vi "GVSResize Panel Child.vi"(8 "spliter array":refnum<vi>[](array[refnum]), 9 "SubPanel array":refnum<vi>[](array[refnum]), 10 "DataView Array Idx":i32) -> ()   [LabVIEW 2013]
uses:
  GVSNew View Global.vi
panel:
  in  "cur_sp_hei":i32
  in  "cur_sp_wid":i32
  in  "cur_sp_ypos":i32
  in  "cur_sp_xpos":i32
  in  "sp_mUp_hei":i32
  in  "sp_mUp_wid":i32
  in  "sp_mUp_ypos":i32
  in  "sp_mUp_xpos":i32
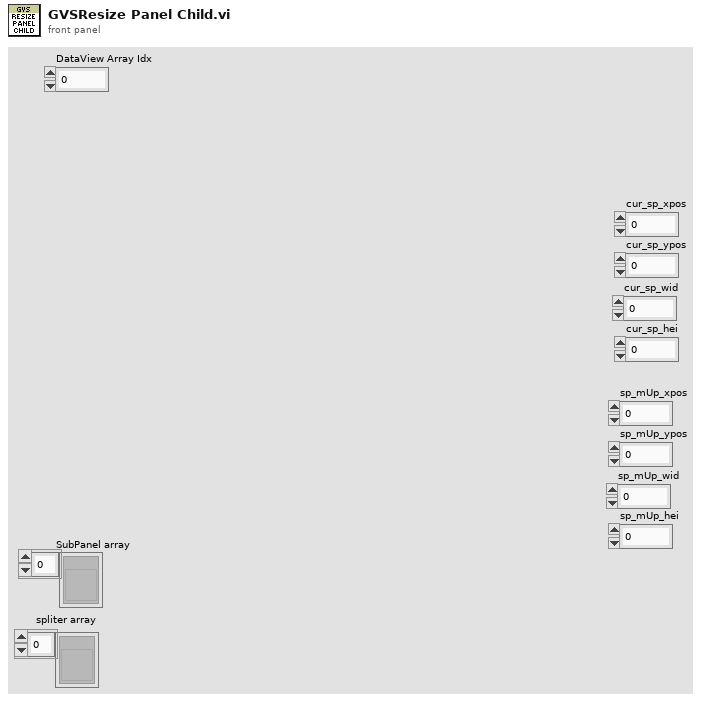
[diagram p1: front panel]
types:
  T1 = typedef "Graph Main Info Cluster.ctl" = cluster{"Selected_BarIdx":i32, "Selected_PanelIdx":i32, "Graph Main VIRef":refnum<vi>, "ToolBarClick":bool, "Spliter Ref Array":refnum<vi>[], "Panel Ref Array":refnum<vi>[], "Spliter_matrix":i32[][], "Panel_matrix":i32[][], "child_spliterIdx_matrix":i32[][], "split_pos_matrix":i32[][], "Title State":bool, "sQueueName":string, "Frame nID":i32, "Graph VIRef Array":cluster{"Graph VIRef":refnum<vi>, "Panel Idx":i32, "Frame VIRef":refnum<vi>, "Icon Ring":i32, "Graph Type":string}[], "View Type":string}
  T2 = typedef "LVPositionTypeDef.ctl" = cluster{"Left":i32, "Top":i32}
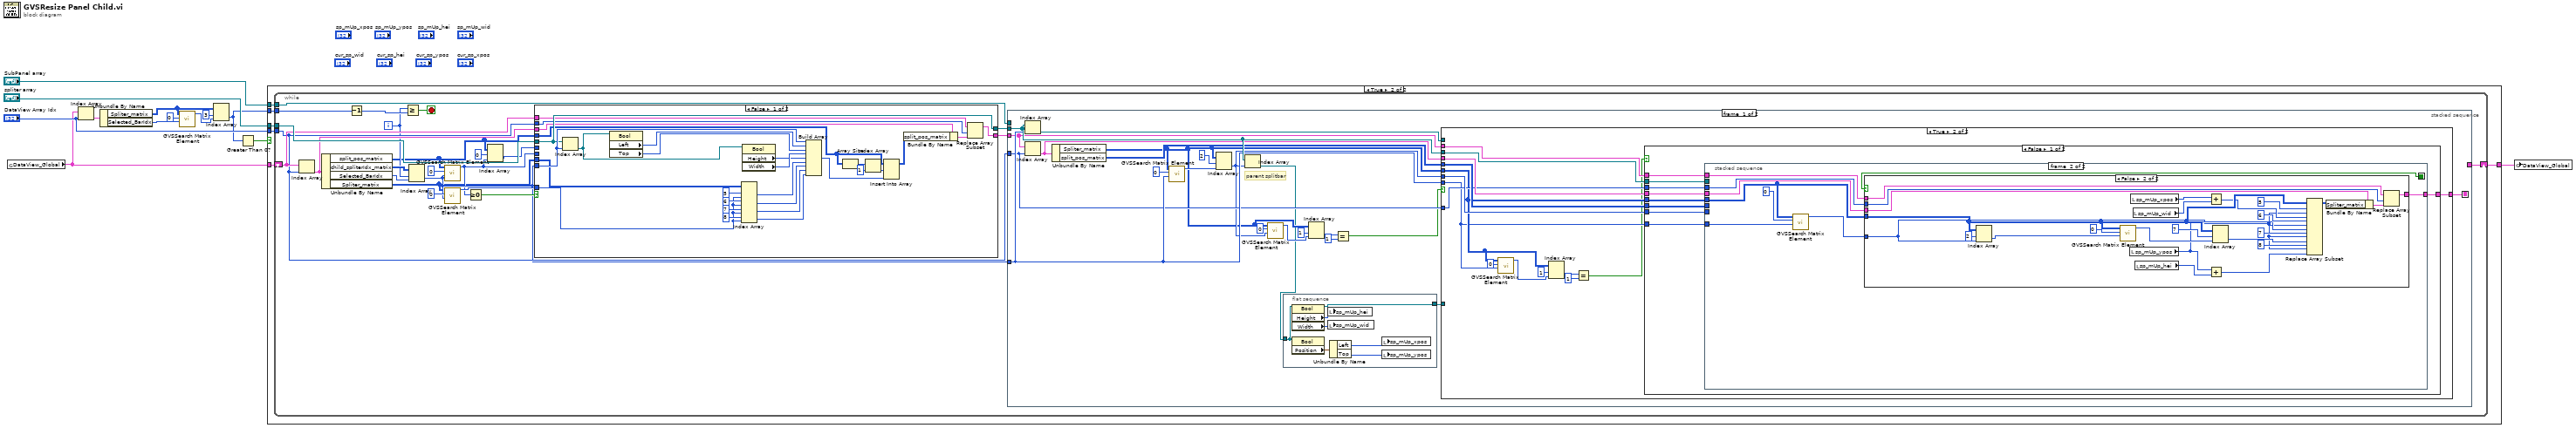
[diagram p0: block diagram]
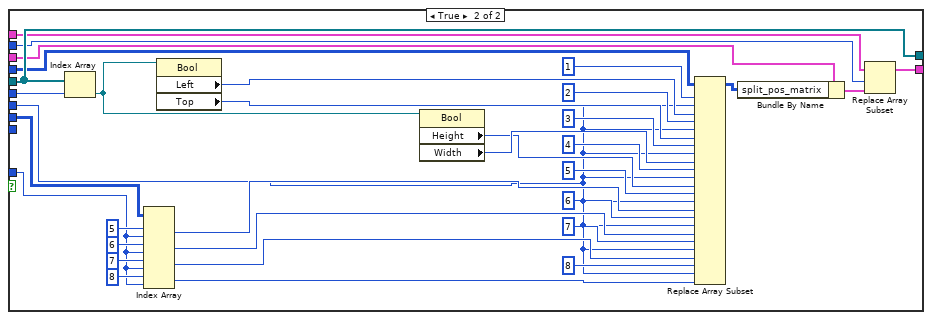
[diagram p3: hidden frame]
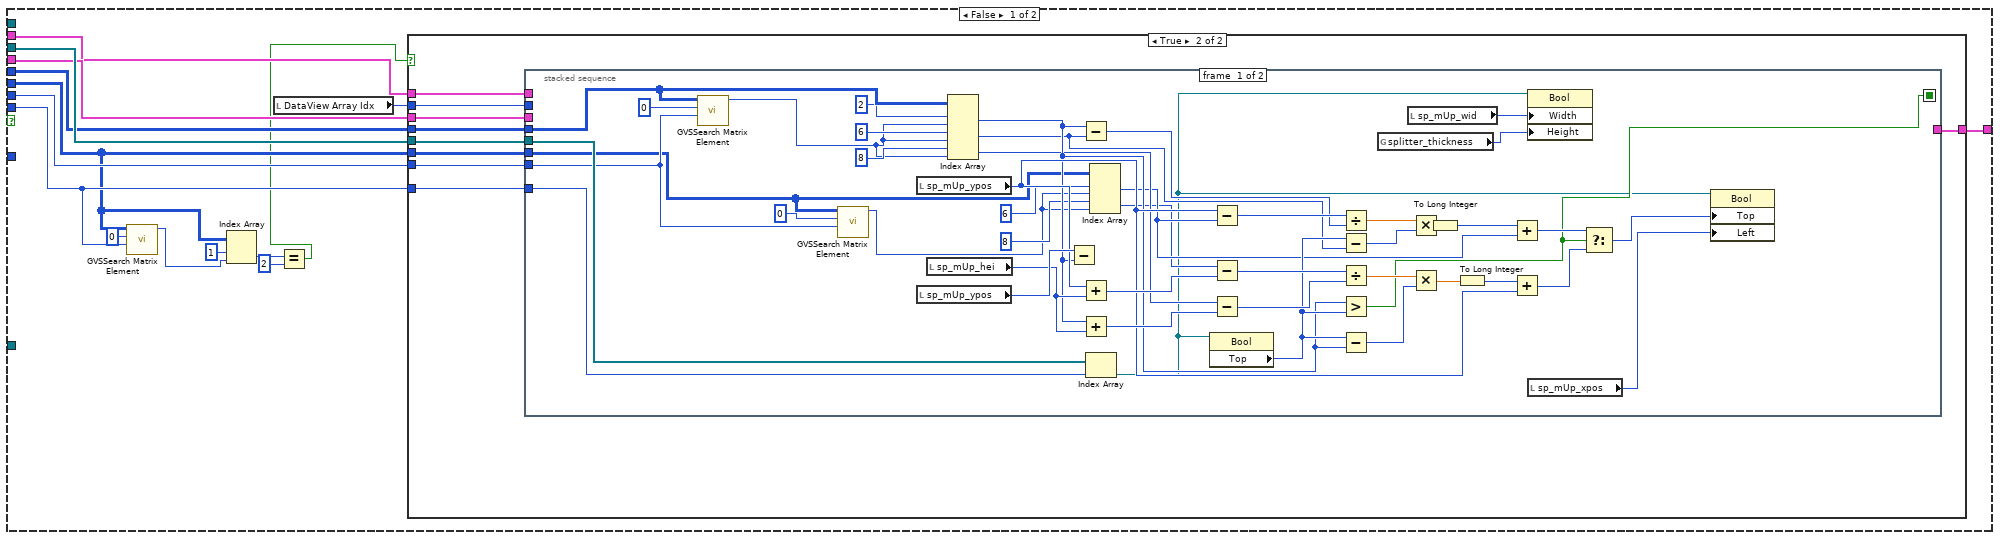
[diagram p4: hidden frame]
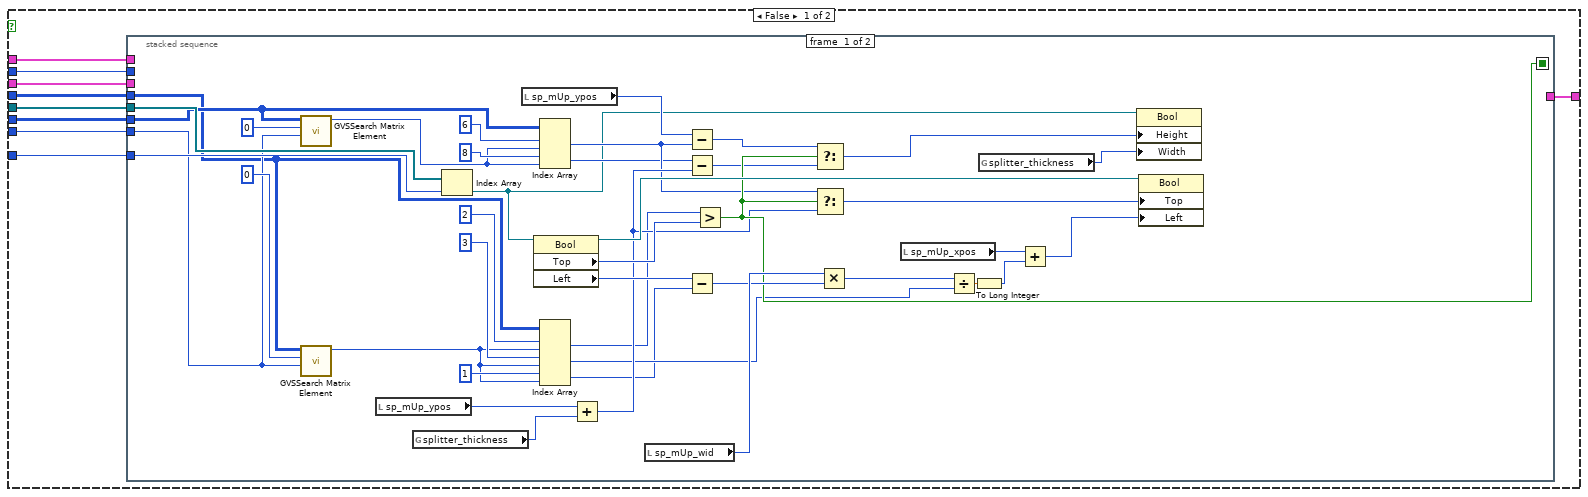
[diagram p5: hidden frame]
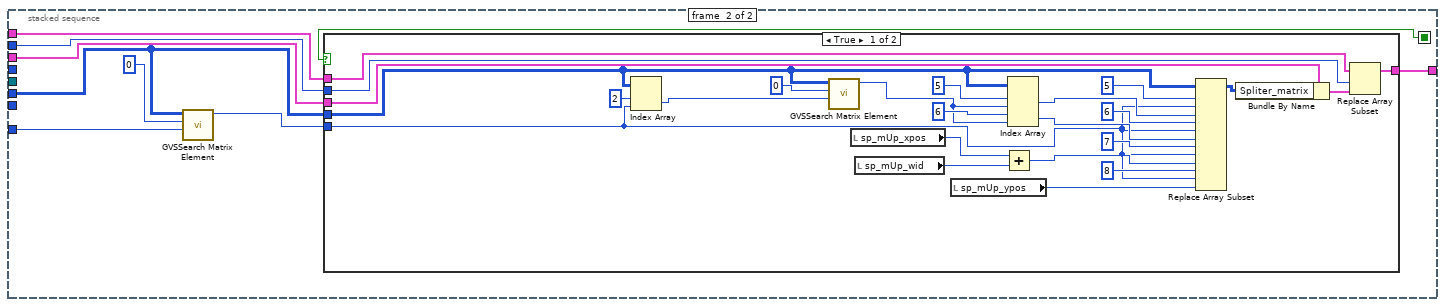
[diagram p6: hidden frame]
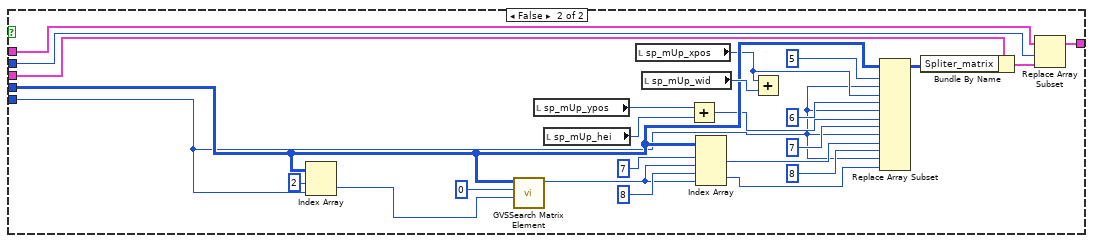
[diagram p7: hidden frame]
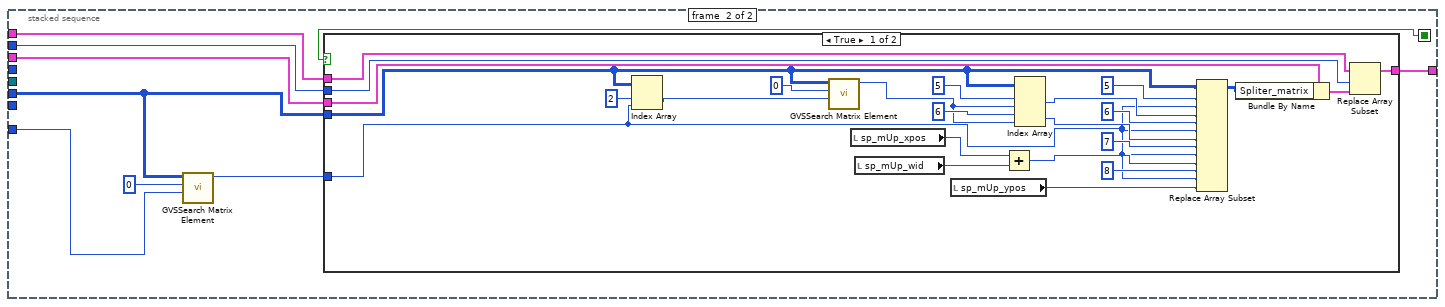
[diagram p8: hidden frame]
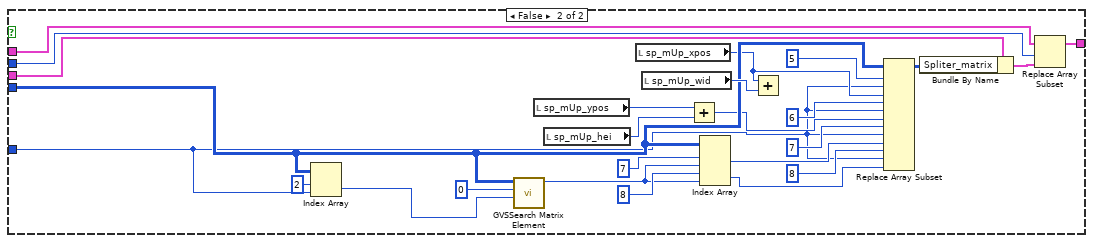
[diagram p9: hidden frame]
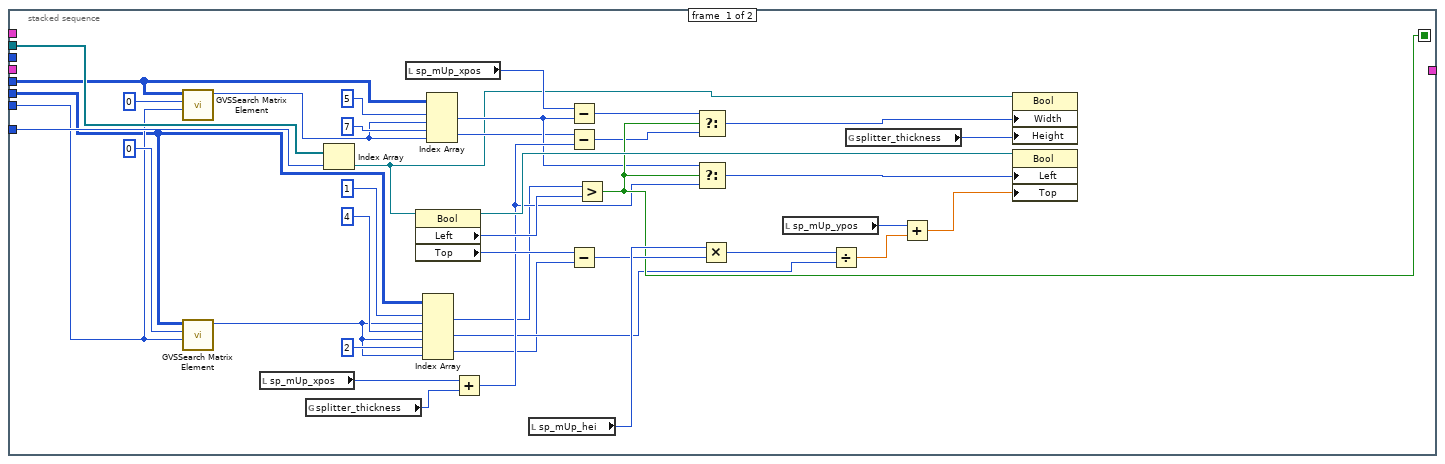
[diagram p10: hidden frame]
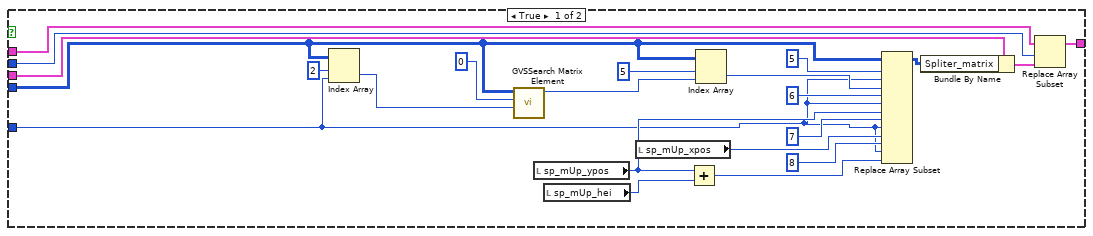
[diagram p11: hidden frame]
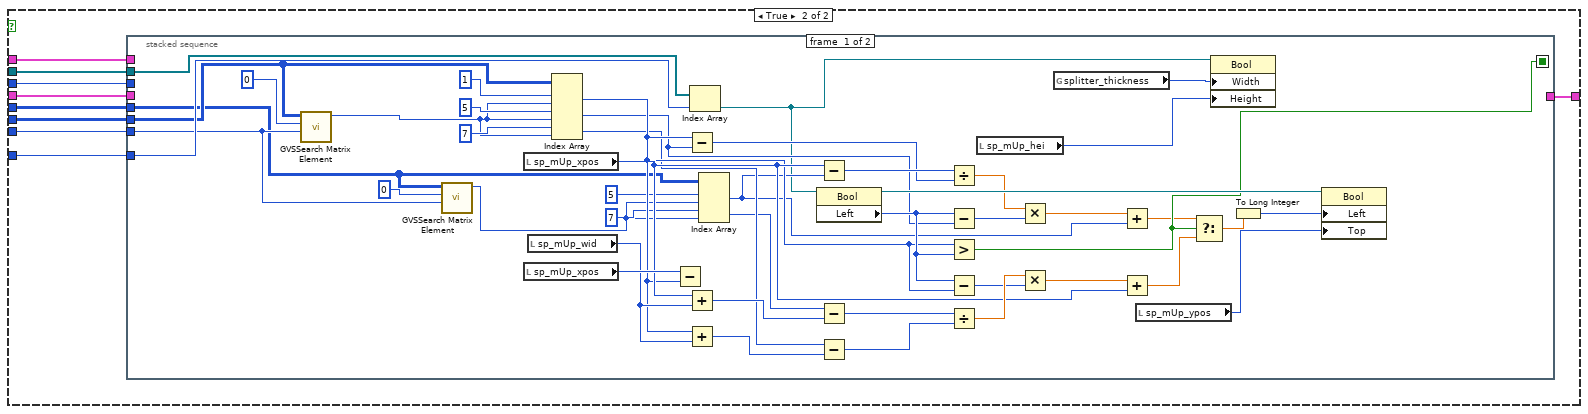
[diagram p12: hidden frame]
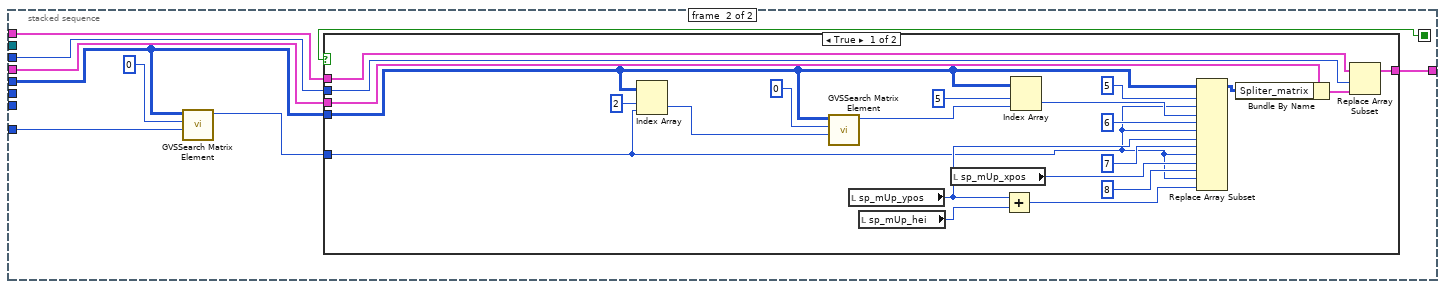
[diagram p13: hidden frame]
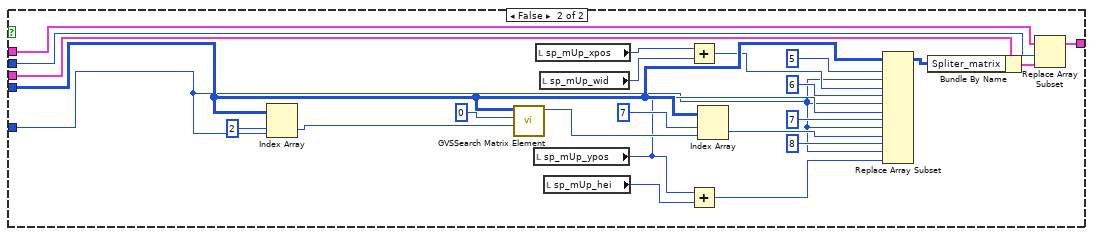
[diagram p14: hidden frame]
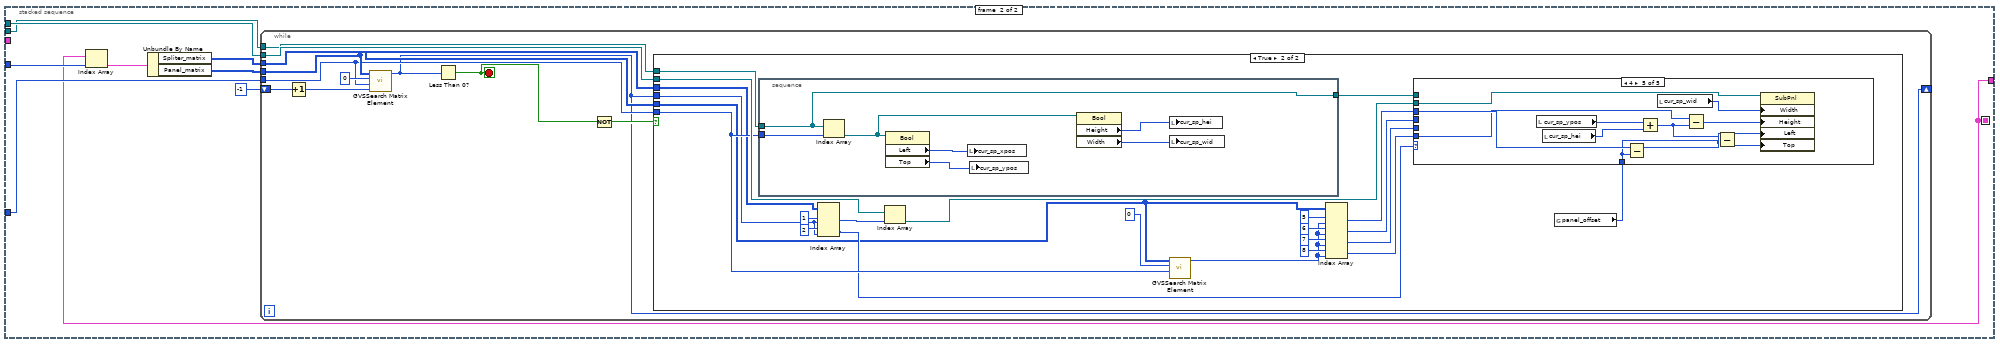
[diagram p15: hidden frame]
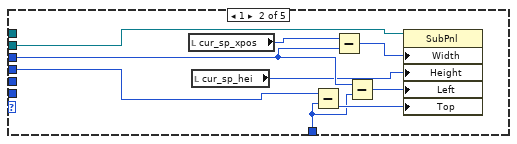
[diagram p18: hidden frame]
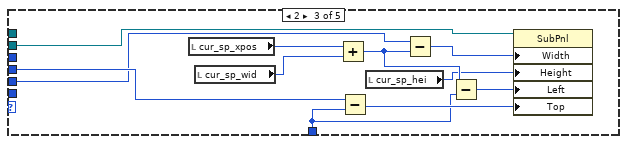
[diagram p19: hidden frame]
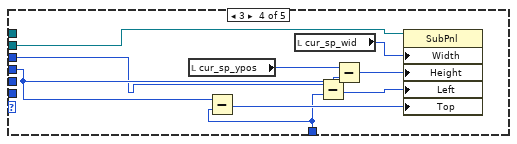
[diagram p20: hidden frame]
diagram:
  n1 = global read "GVSNew View Global.vi" "DataView_Global"() -> (w7:T1[])
  n2 = Index Array(array=w7, index="DataView Array Idx") -> (element=w10:T1)
  n3 = Unbundle By Name(w10) -> ("Spliter_matrix"=w4:i32[][], "Selected_BarIdx"=w9:i32)
  n4 = call "GVSSearch Matrix Element.vi"("element"=w9, "index (row)"=0, "matrix in"=w4) -> ("index of element"=w2:i32)  [unwired: 8 in]
  n5 = Index Array(array=w4, index (row)=3, index (col)=w2) -> (element=w1:i32)
  n6 = Greater Than 0?(x=w1) -> (x > 0?=w5:bool)
  n7 = case shown="True" w5 {
    tunnel: "spliter array" -> [_ w20]
    tunnel: "SubPanel array" -> [_ w19]
    tunnel: "DataView Array Idx" -> [_ w18]
    tunnel: w1 -> [_ w17]
    tunnel: w7 -> [w14 w16]
    tunnel: [w14 w15] -> w6
    frame False {
    }
    frame True {
      n8 = while {
        tunnel: w20 -> [w41]
        tunnel: w17 -> [w30]
        tunnel: w19 -> [w39]
        tunnel: w18 -> [w31]
        shift-right: [w32] -> w15
        shift-left: w16 -> [w34]
        i -> [w28]
        stop <- w42 stop-if-true
        n9 = Index Array(array=w34, index=w31) -> (element=w38:T1)
        n10 = Unbundle By Name(w38) -> ("split_pos_matrix"=w24:i32[][], "child_spliterIdx_matrix"=w29:i32[][], "Selected_BarIdx"=w27:i32, "Spliter_matrix"=w21:i32[][])
        n11 = Decrement(x=w30) -> (x-1=w43:i32)
        n12 = Greater Or Equal?(x=w28, y=w43) -> (x >= y?=w42:bool)
        n13 = Index Array(array=w29, index (row)=w28, index (col)=w27) -> (element=w26:i32)
        n14 = call "GVSSearch Matrix Element.vi"("element"=w26, "index (row)"=0, "matrix in"=w24) -> ("index of element"=w23:i32)  [unwired: 8 in]
        n15 = call "GVSSearch Matrix Element.vi"("element"=w26, "index (row)"=0, "matrix in"=w21) -> ("index of element"=w36:i32)  [unwired: 8 in]
        n16 = Greater Or Equal To 0?(x=w23) -> (x >= 0?=w44:bool)
        n17 = Index Array(array=w24, index (row)=0, index (col)=w23) -> (element=w22:i32)
        n18 = case shown="False" w44 {
          tunnel: w23 -> [_ w76]
          tunnel: w26 -> [w72 _]
          tunnel: w41 -> [w67 w104]
          tunnel: w22 -> [_ w105]
          tunnel: [w67 w104] -> w40
          tunnel: w36 -> [w57 w93]
          tunnel: w21 -> [w56 w94]
          tunnel: w24 -> [w48 w92]
          tunnel: w31 -> [w65 w102]
          tunnel: w38 -> [w64 w101]
          tunnel: w34 -> [w63 w100]
          tunnel: [w62 w99] -> w33
          frame False {
            n19 = Index Array(array=w67, index=w72) -> (element=w45:refnum<vi>)
            n20 = property class="Bool"(reference=w45) -> ("Left"=w71:i32, "Top"=w70:i32)  [unwired: 1 in, 2 out]
            n21 = Index Array(array=w56, index (row) #1=5 ("index (row)"), index (col) #1=w57, index (row) #2=6 ("index (row)"), index (col) #2=w57, index (row) #3=7 ("index (row)"), index (col) #3=w57, index (row) #4=8 ("index (row)"), index (col) #4=w57) -> (element #1=w55:i32, element #2=w54:i32, element #3=w53:i32, element #4=w52:i32)
            n22 = property class="Bool"(reference=w45) -> ("Height"=w68:u32, "Width"=w69:u32)  [unwired: 1 in, 2 out]
            n23 = Build Array(w72, w71, w70, w69, w68, w55, w54, w53, w52) -> (w47:u32[])
            n24 = Array Size(array=w48) -> (size(s)=w51:i32[])
            n25 = Index Array(array=w51, index=1) -> (element=w49:i32)
            n26 = Insert Into Array(array=w48, index (col)=w49, new element=w47) -> (w46:i32[][])  [unwired: 1 in]
            n27 = Bundle By Name(cluster=w64, "split_pos_matrix"=w46) -> (w66:T1)
            n28 = Replace Array Subset(array=w63, new element=w66, index=w65) -> (w62:T1[])
          }
          frame True {
            n29 = Index Array(array=w104, index=w105) -> (element=w73:refnum<vi>)
            n30 = Index Array(array=w94, index (row) #1=5 ("index (row)"), index (col) #1=w93, index (row) #2=6 ("index (row)"), index (col) #2=w93, index (row) #3=7 ("index (row)"), index (col) #3=w93, index (row) #4=8 ("index (row)"), index (col) #4=w93) -> (element #1=w82:i32, element #2=w80:i32, element #3=w78:i32, element #4=w75:i32)
            n31 = property class="Bool"(reference=w73) -> ("Left"=w90:i32, "Top"=w88:i32)  [unwired: 1 in, 2 out]
            n32 = property class="Bool"(reference=w73) -> ("Height"=w84:u32, "Width"=w86:u32)  [unwired: 1 in, 2 out]
            n33 = Replace Array Subset(array=w92, new element #1=w90, index (row) #1=1 ("disabled index (row)"), index (col) #1=w76, new element #2=w88, index (row) #2=2 ("disabled index (row)"), index (col) #2=w76, new element #3=w86, index (row) #3=3 ("disabled index (row)"), index (col) #3=w76, new element #4=w84, index (row) #4=4 ("disabled index (row)"), index (col) #4=w76, new element #5=w82, index (row) #5=5 ("disabled index (row)"), index (col) #5=w76, new element #6=w80, index (row) #6=6 ("disabled index (row)"), index (col) #6=w76, new element #7=w78, index (row) #7=7 ("disabled index (row)"), index (col) #7=w76, new element #8=w75, index (row) #8=8 ("disabled index (row)"), index (col) #8=w76) -> (w74:i32[][])
            n34 = Bundle By Name(cluster=w101, "split_pos_matrix"=w74) -> (w103:T1)
            n35 = Replace Array Subset(array=w100, new element=w103, index=w102) -> (w99:T1[])
          }
        }
        n36 = stacked-sequence {
          seq-local: [w119 _] -> [_ w595]
          tunnel: w40 -> [w125 w601]
          tunnel: w26 -> [w121 w603]
          tunnel: w39 -> [_ w602]
          tunnel: w31 -> [w118 w598]
          tunnel: w33 -> [w120 _]
          tunnel: [_ w595] -> w32
          frame #0 {
            # "parent splitbar"
            n37 = Index Array(array=w125, index=w121) -> (element=w126:refnum<vi>)
            n38 = Index Array(array=w120, index=w118) -> (element=w123:T1)
            n39 = Unbundle By Name(w123) -> ("Spliter_matrix"=w113:i32[][], "split_pos_matrix"=w124:i32[][])
            n40 = call "GVSSearch Matrix Element.vi"("element"=w121, "index (row)"=0, "matrix in"=w113) -> ("index of element"=w116:i32)  [unwired: 8 in]
            n41 = Index Array(array=w113, index (row)=2, index (col)=w116) -> (element=w114:i32)
            n42 = Index Array(array=w125, index=w114) -> (element=w107:refnum<vi>)
            n43 = call "GVSSearch Matrix Element.vi"("element"=w114, "index (row)"=0, "matrix in"=w113) -> ("index of element"=w111:i32)  [unwired: 8 in]
            n44 = flat-sequence {
              tunnel: w107 -> [w128]
              tunnel: [w127] -> w106
              frame #0 {
                n45 = property class="Bool"(reference=w128) -> (reference out=w127:refnum<vi>, "Height"=w130:u32, "Width"=w129:u32)  [unwired: 1 in, 1 out]
                n46 = property class="Bool"(reference=w128) -> ("Position"=w133:T2)  [unwired: 1 in, 2 out]
                n47 = local write "sp_mUp_hei"(w130) -> ()
                n48 = local write "sp_mUp_wid"(w129) -> ()
                n49 = Unbundle By Name(w133) -> ("Left"=w132:i32, "Top"=w131:i32)
                n50 = local write "sp_mUp_xpos"(w132) -> ()
                n51 = local write "sp_mUp_ypos"(w131) -> ()
              }
            }
            n52 = Index Array(array=w113, index (row)=1, index (col)=w111) -> (element=w110:i32)
            n53 = Equal?(x=w110, y=1) -> (x = y?=w108:bool)
            n54 = case shown="True" w108 {
              tunnel: w126 -> [_ _]
              tunnel: w114 -> [w148 w382]
              tunnel: w125 -> [w147 w381]
              tunnel: w121 -> [w141 w369]
              tunnel: w124 -> [w146 w380]
              tunnel: w113 -> [w136 w370]
              tunnel: w123 -> [w145 w379]
              tunnel: w120 -> [w143 w378]
              tunnel: [w142 w377] -> w119
              tunnel: w118 -> [_ w376]
              tunnel: w106 -> [_ _]
              frame False {
                n55 = call "GVSSearch Matrix Element.vi"("element"=w141, "index (row)"=0, "matrix in"=w136) -> ("index of element"=w135:i32)  [unwired: 8 in]
                n56 = Index Array(array=w136, index (row)=1, index (col)=w135) -> (element=w138:i32)
                n57 = local read "DataView Array Idx"() -> (w144:i32)
                n58 = Equal?(x=w138, y=2) -> (x = y?=w134:bool)
                n59 = case shown="True" w134 {
                  tunnel: w148 -> [w155 w262]
                  tunnel: w147 -> [w157 w263]
                  tunnel: w141 -> [w156 w264]
                  tunnel: w146 -> [w154 w261]
                  tunnel: w136 -> [w153 w260]
                  tunnel: w145 -> [w152 w259]
                  tunnel: w144 -> [w151 w258]
                  tunnel: w143 -> [w150 w257]
                  tunnel: [w149 w256] -> w142
                  frame False {
                    n60 = stacked-sequence {
                      seq-local: [w184 _] -> [_ w206]
                      tunnel: w157 -> [w196 _]
                      tunnel: w156 -> [w195 w201]
                      tunnel: w155 -> [w176 _]
                      tunnel: w154 -> [w169 _]
                      tunnel: w153 -> [w175 w203]
                      tunnel: w152 -> [_ w205]
                      tunnel: w151 -> [_ w204]
                      tunnel: w150 -> [_ w199]
                      tunnel: [_ w198] -> w149
                      frame #0 {
                        n61 = call "GVSSearch Matrix Element.vi"("element"=w176, "index (row)"=0, "matrix in"=w175) -> ("index of element"=w172:i32)  [unwired: 8 in]
                        n62 = call "GVSSearch Matrix Element.vi"("element"=w176, "index (row)"=0, "matrix in"=w169) -> ("index of element"=w165:i32)  [unwired: 8 in]
                        n63 = local read "sp_mUp_ypos"() -> (w194:i32)
                        n64 = global read "GVSNew View Global.vi" "splitter_thickness"() -> (w158:u32)
                        n65 = Index Array(array=w196, index=w195) -> (element=w161:refnum<vi>)
                        n66 = local read "sp_mUp_ypos"() -> (w182:i32)
                        n67 = property class="Bool"(reference=w161) -> (reference out=w197:refnum<vi>, "Top"=w183:i32, "Left"=w186:i32)  [unwired: 1 in, 1 out]
                        n68 = Index Array(array=w175, index (row) #1=6 ("index (row)"), index (col) #1=w172, index (row) #2=8 ("index (row)"), index (col) #2=w172) -> (element #1=w171:i32, element #2=w170:i32)
                        n69 = Index Array(array=w169, index (row) #1=2 ("index (row)"), index (col) #1=w165, index (row) #2=3 ("index (row)"), index (col) #2=w165, index (row) #3=1 ("index (row)"), index (col) #3=w165) -> (element #1=w164:i32, element #2=w163:i32, element #3=w162:i32)
                        n70 = Add(x=w194, y=w158) -> (x+y=w180:u32)
                        n71 = local read "sp_mUp_wid"() -> (w191:i32)
                        n72 = Subtract(x=w182, y=w171) -> (x-y=w181:i32)
                        n73 = Subtract(x=w170, y=w180) -> (x-y=w179:u32)
                        n74 = Subtract(x=w186, y=w162) -> (x-y=w185:i32)
                        n75 = Greater?(x=w164, y=w183) -> (0:w184:bool)
                        n76 = Select(t=w181, s=w184, f=w179) -> (s? t:f=w192:u32)
                        n77 = Select(t=w171, s=w184, f=w180) -> (s? t:f=w193:u32)
                        n78 = Multiply(x=w191, y=w185) -> (x*y=w190:i32)
                        n79 = local read "sp_mUp_xpos"() -> (w189:i32)
                        n80 = Divide(x=w190, y=w163) -> (x/y=w188:dbl)
                        n81 = To Long Integer(number=w188) -> (32bit integer=w160:i32)
                        n82 = global read "GVSNew View Global.vi" "splitter_thickness"() -> (w159:u32)
                        n83 = Add(x=w189, y=w160) -> (x+y=w187:i32)
                        n84 = property class="Bool"(reference=w161, "Height"=w192, "Width"=w159) -> ()  [unwired: 1 in, 2 out]
                        n85 = property class="Bool"(reference=w197, "Top"=w193, "Left"=w187) -> ()  [unwired: 1 in, 2 out]
                      }
                      frame #1 {
                        n86 = call "GVSSearch Matrix Element.vi"("element"=w201, "index (row)"=0, "matrix in"=w203) -> ("index of element"=w200:i32)  [unwired: 8 in]
                        n87 = case shown="True" w206 {
                          tunnel: w200 -> [w209 w233]
                          tunnel: w203 -> [w217 w241]
                          tunnel: w205 -> [w227 w251]
                          tunnel: w204 -> [w226 w250]
                          tunnel: w199 -> [w224 w248]
                          tunnel: [w223 w247] -> w198
                          frame True {
                            n88 = Index Array(array=w217, index (row)=2, index (col)=w209) -> (element=w221:i32)
                            n89 = call "GVSSearch Matrix Element.vi"("element"=w221, "index (row)"=0, "matrix in"=w217) -> ("index of element"=w218:i32)  [unwired: 8 in]
                            n90 = local read "sp_mUp_xpos"() -> (w229:i32)
                            n91 = local read "sp_mUp_wid"() -> (w230:i32)
                            n92 = local read "sp_mUp_ypos"() -> (w208:i32)
                            n93 = Add(x=w229, y=w230) -> (x+y=w211:i32)
                            n94 = Index Array(array=w217, index (row) #1=5 ("index (row)"), index (col) #1=w218, index (row) #2=6 ("index (row)"), index (col) #2=w218) -> (element #1=w215:i32, element #2=w213:i32)
                            n95 = Replace Array Subset(array=w217, new element #1=w215, index (row) #1=5 ("disabled index (row)"), index (col) #1=w209, new element #2=w213, index (row) #2=6 ("disabled index (row)"), index (col) #2=w209, new element #3=w211, index (row) #3=7 ("disabled index (row)"), index (col) #3=w209, new element #4=w208, index (row) #4=8 ("disabled index (row)"), index (col) #4=w209) -> (w207:i32[][])
                            n96 = Bundle By Name(cluster=w227, "Spliter_matrix"=w207) -> (w228:T1)
                            n97 = Replace Array Subset(array=w224, new element=w228, index=w226) -> (w223:T1[])
                          }
                          frame False {
                            n98 = Index Array(array=w241, index (row)=2, index (col)=w233) -> (element=w245:i32)
                            n99 = call "GVSSearch Matrix Element.vi"("element"=w245, "index (row)"=0, "matrix in"=w241) -> ("index of element"=w242:i32)  [unwired: 8 in]
                            n100 = local read "sp_mUp_ypos"() -> (w254:i32)
                            n101 = local read "sp_mUp_hei"() -> (w255:i32)
                            n102 = local read "sp_mUp_xpos"() -> (w239:i32)
                            n103 = local read "sp_mUp_wid"() -> (w253:i32)
                            n104 = Add(x=w254, y=w255) -> (x+y=w237:i32)
                            n105 = Index Array(array=w241, index (row) #1=7 ("index (row)"), index (col) #1=w242, index (row) #2=8 ("index (row)"), index (col) #2=w242) -> (element #1=w235:i32, element #2=w232:i32)
                            n106 = Add(x=w239, y=w253) -> ()  [unwired: 1 out]
                            n107 = Replace Array Subset(array=w241, new element #1=w239, index (row) #1=5 ("disabled index (row)"), index (col) #1=w233, new element #2=w237, index (row) #2=6 ("disabled index (row)"), index (col) #2=w233, new element #3=w235, index (row) #3=7 ("disabled index (row)"), index (col) #3=w233, new element #4=w232, index (row) #4=8 ("disabled index (row)"), index (col) #4=w233) -> (w231:i32[][])
                            n108 = Bundle By Name(cluster=w251, "Spliter_matrix"=w231) -> (w252:T1)
                            n109 = Replace Array Subset(array=w248, new element=w252, index=w250) -> (w247:T1[])
                          }
                        }
                      }
                    }
                  }
                  frame True {
                    n110 = stacked-sequence {
                      seq-local: [w286 _] -> [_ w318]
                      tunnel: w264 -> [w308 w314]
                      tunnel: w263 -> [w307 _]
                      tunnel: w262 -> [w283 _]
                      tunnel: w261 -> [w282 _]
                      tunnel: w260 -> [w274 w313]
                      tunnel: w259 -> [_ w317]
                      tunnel: w258 -> [_ w316]
                      tunnel: w257 -> [_ w311]
                      tunnel: [_ w310] -> w256
                      frame #0 {
                        n111 = call "GVSSearch Matrix Element.vi"("element"=w283, "index (row)"=0, "matrix in"=w282) -> ("index of element"=w278:i32)  [unwired: 8 in]
                        n112 = call "GVSSearch Matrix Element.vi"("element"=w283, "index (row)"=0, "matrix in"=w274) -> ("index of element"=w271:i32)  [unwired: 8 in]
                        n113 = local read "sp_mUp_ypos"() -> (w291:i32)
                        n114 = local read "sp_mUp_ypos"() -> (w309:i32)
                        n115 = local read "sp_mUp_hei"() -> (w304:i32)
                        n116 = Index Array(array=w282, index (row) #1=2 ("index (row)"), index (col) #1=w278, index (row) #2=6 ("index (row)"), index (col) #2=w278, index (row) #3=8 ("index (row)"), index (col) #3=w278) -> (element #1=w277:i32, element #2=w276:i32, element #3=w275:i32)
                        n117 = Subtract(x=w309, y=w277) -> ()  [unwired: 1 out]
                        n118 = Subtract(x=w277, y=w276) -> (x-y=w298:i32)
                        n119 = Add(x=w291, y=w304) -> (x+y=w292:i32)
                        n120 = Add(x=w277, y=w304) -> (x+y=w293:i32)
                        n121 = Index Array(array=w307, index=w308) -> (element=w268:refnum<vi>)
                        n122 = Index Array(array=w274, index (row) #1=6 ("index (row)"), index (col) #1=w271, index (row) #2=8 ("index (row)"), index (col) #2=w271) -> (element #1=w270:i32, element #2=w269:i32)
                        n123 = property class="Bool"(reference=w268) -> ("Top"=w290:i32)  [unwired: 1 in, 2 out]
                        n124 = Subtract(x=w291, y=w270) -> (x-y=w299:i32)
                        n125 = Subtract(x=w269, y=w292) -> (x-y=w303:i32)
                        n126 = Subtract(x=w275, y=w293) -> (x-y=w302:i32)
                        n127 = Divide(x=w299, y=w298) -> (x/y=w297:dbl)
                        n128 = Subtract(x=w290, y=w276) -> (x-y=w296:i32)
                        n129 = Divide(x=w303, y=w302) -> (x/y=w301:dbl)
                        n130 = Greater?(x=w277, y=w290) -> (0:w286:bool)
                        n131 = Subtract(x=w290, y=w277) -> (x-y=w294:i32)
                        n132 = global read "GVSNew View Global.vi" "splitter_thickness"() -> (w265:u32)
                        n133 = local read "sp_mUp_wid"() -> (w306:i32)
                        n134 = Multiply(x=w297, y=w296) -> (x*y=w295:dbl)
                        n135 = Multiply(x=w301, y=w294) -> (x*y=w300:dbl)
                        n136 = To Long Integer(number=w295) -> (32bit integer=w267:i32)
                        n137 = To Long Integer(number=w300) -> (32bit integer=w266:i32)
                        n138 = Add(x=w267, y=w270) -> (x+y=w289:i32)
                        n139 = Add(x=w266, y=w291) -> (x+y=w288:i32)
                        n140 = property class="Bool"(reference=w268, "Width"=w306, "Height"=w265) -> ()  [unwired: 1 in, 2 out]
                        n141 = local read "sp_mUp_xpos"() -> (w305:i32)
                        n142 = Select(t=w289, s=w286, f=w288) -> (s? t:f=w287:i32)
                        n143 = property class="Bool"(reference=w268, "Top"=w287, "Left"=w305) -> ()  [unwired: 1 in, 2 out]
                      }
                      frame #1 {
                        n144 = call "GVSSearch Matrix Element.vi"("element"=w314, "index (row)"=0, "matrix in"=w313) -> ("index of element"=w312:i32)  [unwired: 8 in]
                        n145 = case shown="True" w318 {
                          tunnel: w312 -> [w320 w344]
                          tunnel: w313 -> [w329 w353]
                          tunnel: w317 -> [w339 w363]
                          tunnel: w316 -> [w338 w362]
                          tunnel: w311 -> [w336 w360]
                          tunnel: [w335 w359] -> w310
                          frame True {
                            n146 = Index Array(array=w329, index (row)=2, index (col)=w320) -> (element=w334:i32)
                            n147 = call "GVSSearch Matrix Element.vi"("element"=w334, "index (row)"=0, "matrix in"=w329) -> ("index of element"=w330:i32)  [unwired: 8 in]
                            n148 = local read "sp_mUp_xpos"() -> (w341:i32)
                            n149 = local read "sp_mUp_wid"() -> (w342:i32)
                            n150 = local read "sp_mUp_ypos"() -> (w319:i32)
                            n151 = Add(x=w341, y=w342) -> (x+y=w322:i32)
                            n152 = Index Array(array=w329, index (row) #1=5 ("index (row)"), index (col) #1=w330, index (row) #2=6 ("index (row)"), index (col) #2=w330) -> (element #1=w326:i32, element #2=w324:i32)
                            n153 = Replace Array Subset(array=w329, new element #1=w326, index (row) #1=5 ("disabled index (row)"), index (col) #1=w320, new element #2=w324, index (row) #2=6 ("disabled index (row)"), index (col) #2=w320, new element #3=w322, index (row) #3=7 ("disabled index (row)"), index (col) #3=w320, new element #4=w319, index (row) #4=8 ("disabled index (row)"), index (col) #4=w320) -> (w328:i32[][])
                            n154 = Bundle By Name(cluster=w339, "Spliter_matrix"=w328) -> (w340:T1)
                            n155 = Replace Array Subset(array=w336, new element=w340, index=w338) -> (w335:T1[])
                          }
                          frame False {
                            n156 = Index Array(array=w353, index (row)=2, index (col)=w344) -> (element=w357:i32)
                            n157 = call "GVSSearch Matrix Element.vi"("element"=w357, "index (row)"=0, "matrix in"=w353) -> ("index of element"=w354:i32)  [unwired: 8 in]
                            n158 = local read "sp_mUp_ypos"() -> (w366:i32)
                            n159 = local read "sp_mUp_hei"() -> (w367:i32)
                            n160 = local read "sp_mUp_xpos"() -> (w350:i32)
                            n161 = local read "sp_mUp_wid"() -> (w365:i32)
                            n162 = Add(x=w366, y=w367) -> (x+y=w348:i32)
                            n163 = Index Array(array=w353, index (row) #1=7 ("index (row)"), index (col) #1=w354, index (row) #2=8 ("index (row)"), index (col) #2=w354) -> (element #1=w346:i32, element #2=w343:i32)
                            n164 = Add(x=w350, y=w365) -> ()  [unwired: 1 out]
                            n165 = Replace Array Subset(array=w353, new element #1=w350, index (row) #1=5 ("disabled index (row)"), index (col) #1=w344, new element #2=w348, index (row) #2=6 ("disabled index (row)"), index (col) #2=w344, new element #3=w346, index (row) #3=7 ("disabled index (row)"), index (col) #3=w344, new element #4=w343, index (row) #4=8 ("disabled index (row)"), index (col) #4=w344) -> (w352:i32[][])
                            n166 = Bundle By Name(cluster=w363, "Spliter_matrix"=w352) -> (w364:T1)
                            n167 = Replace Array Subset(array=w360, new element=w364, index=w362) -> (w359:T1[])
                          }
                        }
                      }
                    }
                  }
                }
              }
              frame True {
                n168 = call "GVSSearch Matrix Element.vi"("element"=w369, "index (row)"=0, "matrix in"=w370) -> ("index of element"=w371:i32)  [unwired: 8 in]
                n169 = Index Array(array=w370, index (row)=1, index (col)=w371) -> (element=w373:i32)
                n170 = Equal?(x=w373, y=1) -> (x = y?=w368:bool)
                n171 = case shown="False" w368 {
                  tunnel: w382 -> [w390 w494]
                  tunnel: w381 -> [w391 w493]
                  tunnel: w369 -> [w389 w492]
                  tunnel: w380 -> [w388 w491]
                  tunnel: w370 -> [w387 w490]
                  tunnel: w379 -> [w386 w489]
                  tunnel: w376 -> [w385 w488]
                  tunnel: w378 -> [w384 w487]
                  tunnel: [w383 w486] -> w377
                  frame False {
                    n172 = stacked-sequence {
                      seq-local: [w416 _] -> [_ w439]
                      tunnel: w391 -> [w430 _]
                      tunnel: w390 -> [w409 _]
                      tunnel: w389 -> [w429 w434]
                      tunnel: w388 -> [w408 _]
                      tunnel: w387 -> [w400 w436]
                      tunnel: w386 -> [_ w438]
                      tunnel: w385 -> [_ w437]
                      tunnel: w384 -> [_ w432]
                      tunnel: [_ w431] -> w383
                      frame #0 {
                        n173 = call "GVSSearch Matrix Element.vi"("element"=w409, "index (row)"=0, "matrix in"=w400) -> ("index of element"=w397:i32)  [unwired: 8 in]
                        n174 = call "GVSSearch Matrix Element.vi"("element"=w409, "index (row)"=0, "matrix in"=w408) -> ("index of element"=w404:i32)  [unwired: 8 in]
                        n175 = local read "sp_mUp_xpos"() -> (w426:i32)
                        n176 = global read "GVSNew View Global.vi" "splitter_thickness"() -> (w392:u32)
                        n177 = Index Array(array=w430, index=w429) -> (element=w394:refnum<vi>)
                        n178 = local read "sp_mUp_xpos"() -> (w415:i32)
                        n179 = property class="Bool"(reference=w394) -> (reference out=w428:refnum<vi>, "Left"=w427:i32, "Top"=w424:i32)  [unwired: 1 in, 1 out]
                        n180 = Index Array(array=w408, index (row) #1=1 ("index (row)"), index (col) #1=w404, index (row) #2=4 ("index (row)"), index (col) #2=w404, index (row) #3=2 ("index (row)"), index (col) #3=w404) -> (element #1=w403:i32, element #2=w402:i32, element #3=w401:i32)
                        n181 = Index Array(array=w400, index (row) #1=5 ("index (row)"), index (col) #1=w397, index (row) #2=7 ("index (row)"), index (col) #2=w397) -> (element #1=w396:i32, element #2=w395:i32)
                        n182 = Add(x=w426, y=w392) -> (x+y=w413:u32)
                        n183 = local read "sp_mUp_hei"() -> (w423:i32)
                        n184 = Subtract(x=w415, y=w396) -> (x-y=w414:i32)
                        n185 = Subtract(x=w395, y=w413) -> (x-y=w412:u32)
                        n186 = Subtract(x=w424, y=w401) -> (x-y=w422:i32)
                        n187 = Greater?(x=w403, y=w427) -> (0:w416:bool)
                        n188 = Select(t=w414, s=w416, f=w412) -> (s? t:f=w417:u32)
                        n189 = Select(t=w396, s=w416, f=w413) -> (s? t:f=w425:u32)
                        n190 = Multiply(x=w423, y=w422) -> (x*y=w421:i32)
                        n191 = local read "sp_mUp_ypos"() -> (w420:i32)
                        n192 = Divide(x=w421, y=w402) -> (x/y=w419:dbl)
                        n193 = global read "GVSNew View Global.vi" "splitter_thickness"() -> (w393:u32)
                        n194 = Add(x=w420, y=w419) -> (x+y=w418:dbl)
                        n195 = property class="Bool"(reference=w394, "Width"=w417, "Height"=w393) -> ()  [unwired: 1 in, 2 out]
                        n196 = property class="Bool"(reference=w428, "Left"=w425, "Top"=w418) -> ()  [unwired: 1 in, 2 out]
                      }
                      frame #1 {
                        n197 = call "GVSSearch Matrix Element.vi"("element"=w434, "index (row)"=0, "matrix in"=w436) -> ("index of element"=w433:i32)  [unwired: 8 in]
                        n198 = case shown="False" w439 {
                          tunnel: w433 -> [w441 w464]
                          tunnel: w436 -> [w450 w472]
                          tunnel: w438 -> [w459 w481]
                          tunnel: w437 -> [w458 w480]
                          tunnel: w432 -> [w456 w478]
                          tunnel: [w455 w477] -> w431
                          frame True {
                            n199 = Index Array(array=w450, index (row)=2, index (col)=w441) -> (element=w453:i32)
                            n200 = call "GVSSearch Matrix Element.vi"("element"=w453, "index (row)"=0, "matrix in"=w450) -> ("index of element"=w451:i32)  [unwired: 8 in]
                            n201 = local read "sp_mUp_ypos"() -> (w446:i32)
                            n202 = local read "sp_mUp_hei"() -> (w461:i32)
                            n203 = local read "sp_mUp_xpos"() -> (w444:i32)
                            n204 = Add(x=w446, y=w461) -> (x+y=w442:i32)
                            n205 = Index Array(array=w450, index (row)=5, index (col)=w451) -> (element=w448:i32)
                            n206 = Replace Array Subset(array=w450, new element #1=w448, index (row) #1=5 ("disabled index (row)"), index (col) #1=w441, new element #2=w446, index (row) #2=6 ("disabled index (row)"), index (col) #2=w441, new element #3=w444, index (row) #3=7 ("disabled index (row)"), index (col) #3=w441, new element #4=w442, index (row) #4=8 ("disabled index (row)"), index (col) #4=w441) -> (w440:i32[][])
                            n207 = Bundle By Name(cluster=w459, "Spliter_matrix"=w440) -> (w460:T1)
                            n208 = Replace Array Subset(array=w456, new element=w460, index=w458) -> (w455:T1[])
                          }
                          frame False {
                            n209 = Index Array(array=w472, index (row)=2, index (col)=w464) -> (element=w475:i32)
                            n210 = call "GVSSearch Matrix Element.vi"("element"=w475, "index (row)"=0, "matrix in"=w472) -> ("index of element"=w473:i32)  [unwired: 8 in]
                            n211 = local read "sp_mUp_ypos"() -> (w468:i32)
                            n212 = local read "sp_mUp_xpos"() -> (w484:i32)
                            n213 = local read "sp_mUp_wid"() -> (w483:i32)
                            n214 = local read "sp_mUp_hei"() -> (w485:i32)
                            n215 = Add(x=w484, y=w483) -> (x+y=w470:i32)
                            n216 = Add(x=w468, y=w485) -> (x+y=w463:i32)
                            n217 = Index Array(array=w472, index (row)=7, index (col)=w473) -> (element=w466:i32)
                            n218 = Replace Array Subset(array=w472, new element #1=w470, index (row) #1=5 ("disabled index (row)"), index (col) #1=w464, new element #2=w468, index (row) #2=6 ("disabled index (row)"), index (col) #2=w464, new element #3=w466, index (row) #3=7 ("disabled index (row)"), index (col) #3=w464, new element #4=w463, index (row) #4=8 ("disabled index (row)"), index (col) #4=w464) -> (w462:i32[][])
                            n219 = Bundle By Name(cluster=w481, "Spliter_matrix"=w462) -> (w482:T1)
                            n220 = Replace Array Subset(array=w478, new element=w482, index=w480) -> (w477:T1[])
                          }
                        }
                      }
                    }
                  }
                  frame True {
                    n221 = stacked-sequence {
                      seq-local: [w533 _] -> [_ w548]
                      tunnel: w494 -> [w512 _]
                      tunnel: w493 -> [w539 _]
                      tunnel: w492 -> [w519 w543]
                      tunnel: w491 -> [w511 _]
                      tunnel: w490 -> [w503 w544]
                      tunnel: w489 -> [_ w547]
                      tunnel: w488 -> [_ w546]
                      tunnel: w487 -> [_ w541]
                      tunnel: [_ w540] -> w486
                      frame #0 {
                        n222 = call "GVSSearch Matrix Element.vi"("element"=w512, "index (row)"=0, "matrix in"=w511) -> ("index of element"=w507:i32)  [unwired: 8 in]
                        n223 = call "GVSSearch Matrix Element.vi"("element"=w512, "index (row)"=0, "matrix in"=w503) -> ("index of element"=w500:i32)  [unwired: 8 in]
                        n224 = local read "sp_mUp_xpos"() -> (w515:i32)
                        n225 = local read "sp_mUp_xpos"() -> (w537:i32)
                        n226 = local read "sp_mUp_wid"() -> (w532:i32)
                        n227 = Index Array(array=w511, index (row) #1=1 ("index (row)"), index (col) #1=w507, index (row) #2=5 ("index (row)"), index (col) #2=w507, index (row) #3=7 ("index (row)"), index (col) #3=w507) -> (element #1=w506:i32, element #2=w505:i32, element #3=w504:i32)
                        n228 = Subtract(x=w537, y=w506) -> ()  [unwired: 1 out]
                        n229 = Subtract(x=w506, y=w505) -> (x-y=w525:i32)
                        n230 = Add(x=w515, y=w532) -> (x+y=w516:i32)
                        n231 = Add(x=w506, y=w532) -> (x+y=w517:i32)
                        n232 = Index Array(array=w539, index=w519) -> (element=w497:refnum<vi>)
                        n233 = Index Array(array=w503, index (row) #1=5 ("index (row)"), index (col) #1=w500, index (row) #2=7 ("index (row)"), index (col) #2=w500) -> (element #1=w498:i32, element #2=w499:i32)
                        n234 = property class="Bool"(reference=w497) -> (reference out=w536:refnum<vi>, "Left"=w523:i32)  [unwired: 1 in, 1 out]
                        n235 = Subtract(x=w515, y=w498) -> (x-y=w526:i32)
                        n236 = Subtract(x=w499, y=w516) -> (x-y=w531:i32)
                        n237 = Subtract(x=w504, y=w517) -> (x-y=w530:i32)
                        n238 = Divide(x=w526, y=w525) -> (x/y=w524:dbl)
                        n239 = Subtract(x=w523, y=w505) -> (x-y=w522:i32)
                        n240 = Greater?(x=w506, y=w523) -> (0:w533:bool)
                        n241 = Subtract(x=w523, y=w506) -> (x-y=w518:i32)
                        n242 = Divide(x=w531, y=w530) -> (x/y=w529:dbl)
                        n243 = local read "sp_mUp_hei"() -> (w538:i32)
                        n244 = Multiply(x=w524, y=w522) -> (x*y=w521:dbl)
                        n245 = Multiply(x=w529, y=w518) -> (x*y=w528:dbl)
                        n246 = global read "GVSNew View Global.vi" "splitter_thickness"() -> (w496:u32)
                        n247 = Add(x=w521, y=w498) -> (x+y=w520:dbl)
                        n248 = Add(x=w528, y=w515) -> (x+y=w527:dbl)
                        n249 = local read "sp_mUp_ypos"() -> (w535:i32)
                        n250 = Select(t=w520, s=w533, f=w527) -> (s? t:f=w534:dbl)
                        n251 = property class="Bool"(reference=w497, "Width"=w496, "Height"=w538) -> ()  [unwired: 1 in, 2 out]
                        n252 = To Long Integer(number=w534) -> (32bit integer=w495:i32)
                        n253 = property class="Bool"(reference=w536, "Left"=w495, "Top"=w535) -> ()  [unwired: 1 in, 2 out]
                      }
                      frame #1 {
                        n254 = call "GVSSearch Matrix Element.vi"("element"=w543, "index (row)"=0, "matrix in"=w544) -> ("index of element"=w542:i32)  [unwired: 8 in]
                        n255 = case shown="True" w548 {
                          tunnel: w542 -> [w551 w573]
                          tunnel: w544 -> [w559 w581]
                          tunnel: w547 -> [w568 w590]
                          tunnel: w546 -> [w567 w589]
                          tunnel: w541 -> [w565 w587]
                          tunnel: [w564 w586] -> w540
                          frame True {
                            n256 = Index Array(array=w559, index (row)=2, index (col)=w551) -> (element=w562:i32)
                            n257 = call "GVSSearch Matrix Element.vi"("element"=w562, "index (row)"=0, "matrix in"=w559) -> ("index of element"=w560:i32)  [unwired: 8 in]
                            n258 = local read "sp_mUp_ypos"() -> (w555:i32)
                            n259 = local read "sp_mUp_hei"() -> (w570:i32)
                            n260 = local read "sp_mUp_xpos"() -> (w553:i32)
                            n261 = Add(x=w555, y=w570) -> (x+y=w550:i32)
                            n262 = Index Array(array=w559, index (row)=5, index (col)=w560) -> (element=w557:i32)
                            n263 = Replace Array Subset(array=w559, new element #1=w557, index (row) #1=5 ("disabled index (row)"), index (col) #1=w551, new element #2=w555, index (row) #2=6 ("disabled index (row)"), index (col) #2=w551, new element #3=w553, index (row) #3=7 ("disabled index (row)"), index (col) #3=w551, new element #4=w550, index (row) #4=8 ("disabled index (row)"), index (col) #4=w551) -> (w549:i32[][])
                            n264 = Bundle By Name(cluster=w568, "Spliter_matrix"=w549) -> (w569:T1)
                            n265 = Replace Array Subset(array=w565, new element=w569, index=w567) -> (w564:T1[])
                          }
                          frame False {
                            n266 = Index Array(array=w581, index (row)=2, index (col)=w573) -> (element=w584:i32)
                            n267 = call "GVSSearch Matrix Element.vi"("element"=w584, "index (row)"=0, "matrix in"=w581) -> ("index of element"=w582:i32)  [unwired: 8 in]
                            n268 = local read "sp_mUp_ypos"() -> (w577:i32)
                            n269 = local read "sp_mUp_xpos"() -> (w593:i32)
                            n270 = local read "sp_mUp_wid"() -> (w592:i32)
                            n271 = local read "sp_mUp_hei"() -> (w594:i32)
                            n272 = Add(x=w593, y=w592) -> (x+y=w579:i32)
                            n273 = Add(x=w577, y=w594) -> (x+y=w572:i32)
                            n274 = Index Array(array=w581, index (row)=7, index (col)=w582) -> (element=w575:i32)
                            n275 = Replace Array Subset(array=w581, new element #1=w579, index (row) #1=5 ("disabled index (row)"), index (col) #1=w573, new element #2=w577, index (row) #2=6 ("disabled index (row)"), index (col) #2=w573, new element #3=w575, index (row) #3=7 ("disabled index (row)"), index (col) #3=w573, new element #4=w572, index (row) #4=8 ("disabled index (row)"), index (col) #4=w573) -> (w571:i32[][])
                            n276 = Bundle By Name(cluster=w590, "Spliter_matrix"=w571) -> (w591:T1)
                            n277 = Replace Array Subset(array=w587, new element=w591, index=w589) -> (w586:T1[])
                          }
                        }
                      }
                    }
                  }
                }
              }
            }
          }
          frame #1 {
            n278 = Index Array(array=w595, index=w598) -> (element=w599:T1)
            n279 = Unbundle By Name(w599) -> ("Spliter_matrix"=w596:i32[][], "Panel_matrix"=w597:i32[][])
            n280 = while {
              shift-right: [w604] -> _
              shift-left: -1 -> [w607]
              tunnel: w603 -> [w605]
              tunnel: w602 -> [w614]
              tunnel: w601 -> [w613]
              tunnel: w597 -> [w609]
              tunnel: w596 -> [w610]
              stop <- w612 stop-if-true
              n281 = Increment(x=w607) -> (x+1=w606:i32)
              n282 = call "GVSSearch Matrix Element.vi"("start index"=w606, "element"=w605, "index (row)"=0, "matrix in"=w609) -> ("index of element"=w604:i32)  [unwired: 7 in]
              n283 = Less Than 0?(x=w604) -> (x < 0?=w612:bool)
              n284 = Not(x=w612) -> (.not. x?=w611:bool)
              n285 = case shown="True" w611 {
                tunnel: w604 -> [_ w628]
                tunnel: w614 -> [_ w635]
                tunnel: w613 -> [_ w637]
                tunnel: w605 -> [_ w632]
                tunnel: w610 -> [_ w620]
                tunnel: w609 -> [_ w629]
                frame False {
                }
                frame True {
                  n286 = stacked-sequence {
                    tunnel: w637 -> [w639]
                    tunnel: w632 -> [w640]
                    tunnel: [w639] -> w636
                    frame #0 {
                      n287 = Index Array(array=w639, index=w640) -> (element=w638:refnum<vi>)
                      n288 = property class="Bool"(reference=w638) -> ("Left"=w644:i32, "Top"=w643:i32)  [unwired: 1 in, 2 out]
                      n289 = local write "cur_sp_xpos"(w644) -> ()
                      n290 = local write "cur_sp_ypos"(w643) -> ()
                      n291 = property class="Bool"(reference=w638) -> ("Height"=w642:u32, "Width"=w641:u32)  [unwired: 1 in, 2 out]
                      n292 = local write "cur_sp_hei"(w642) -> ()
                      n293 = local write "cur_sp_wid"(w641) -> ()
                    }
                  }
                  n294 = Index Array(array=w629, index (row) #1=1 ("index (row)"), index (col) #1=w628, index (row) #2=2 ("index (row)"), index (col) #2=w628) -> (element #1=w627:i32, element #2=w626:i32)
                  n295 = Index Array(array=w635, index=w627) -> (element=w634:refnum<vi>)
                  n296 = call "GVSSearch Matrix Element.vi"("element"=w632, "index (row)"=0, "matrix in"=w620) -> ("index of element"=w621:i32)  [unwired: 8 in]
                  n297 = Index Array(array=w620, index (row) #1=5 ("index (row)"), index (col) #1=w621, index (row) #2=6 ("index (row)"), index (col) #2=w621, index (row) #3=7 ("index (row)"), index (col) #3=w621, index (row) #4=8 ("index (row)"), index (col) #4=w621) -> (element #1=w619:i32, element #2=w618:i32, element #3=w617:i32, element #4=w616:i32)
                  n298 = global read "GVSNew View Global.vi" "panel_offset"() -> (w615:i32)
                  n299 = case shown="4" w626 {
                    tunnel: w619 -> [_ w653 _ w666 w682]
                    tunnel: w618 -> [_ w647 w661 w670 _]
                    tunnel: w617 -> [_ _ w660 _ _]
                    tunnel: w616 -> [_ _ _ _ w679]
                    tunnel: w636 -> [_ _ _ _ _]
                    tunnel: w634 -> [_ w649 w664 w673 w684]
                    tunnel: w615 -> [_ w645 w654 w665 w674]
                    frame 0, Default {
                    }
                    frame 1 {
                      n300 = local read "cur_sp_xpos"() -> (w652:i32)
                      n301 = local read "cur_sp_hei"() -> (w650:i32)
                      n302 = Subtract(x=w647, y=w645) -> (x-y=w648:i32)
                      n303 = Subtract(x=w652, y=w653) -> (x-y=w651:i32)
                      n304 = Subtract(x=w653, y=w645) -> (x-y=w646:i32)
                      n305 = property class="SubPnl"(reference=w649, "Width"=w651, "Height"=w650, "Left"=w646, "Top"=w648) -> ()  [unwired: 1 in, 2 out]
                    }
                    frame 2 {
                      n306 = local read "cur_sp_xpos"() -> (w663:i32)
                      n307 = local read "cur_sp_wid"() -> (w662:i32)
                      n308 = Add(x=w663, y=w662) -> (x+y=w659:i32)
                      n309 = Subtract(x=w661, y=w654) -> (x-y=w656:i32)
                      n310 = local read "cur_sp_hei"() -> (w657:i32)
                      n311 = Subtract(x=w660, y=w659) -> (x-y=w658:i32)
                      n312 = Subtract(x=w659, y=w654) -> (x-y=w655:i32)
                      n313 = property class="SubPnl"(reference=w664, "Width"=w658, "Height"=w657, "Left"=w655, "Top"=w656) -> ()  [unwired: 1 in, 2 out]
                    }
                    frame 3 {
                      n314 = local read "cur_sp_ypos"() -> (w671:i32)
                      n315 = Subtract(x=w670, y=w665) -> (x-y=w668:i32)
                      n316 = local read "cur_sp_wid"() -> (w672:i32)
                      n317 = Subtract(x=w666, y=w665) -> (x-y=w667:i32)
                      n318 = Subtract(x=w671, y=w670) -> (x-y=w669:i32)
                      n319 = property class="SubPnl"(reference=w673, "Width"=w672, "Height"=w669, "Left"=w667, "Top"=w668) -> ()  [unwired: 1 in, 2 out]
                    }
                    frame 4 {
                      n320 = local read "cur_sp_ypos"() -> (w681:i32)
                      n321 = local read "cur_sp_hei"() -> (w680:i32)
                      n322 = Subtract(x=w682, y=w674) -> (x-y=w677:i32)
                      n323 = Add(x=w681, y=w680) -> (x+y=w675:i32)
                      n324 = local read "cur_sp_wid"() -> (w683:i32)
                      n325 = Subtract(x=w679, y=w675) -> (x-y=w678:i32)
                      n326 = Subtract(x=w675, y=w674) -> (x-y=w676:i32)
                      n327 = property class="SubPnl"(reference=w684, "Width"=w683, "Height"=w678, "Left"=w677, "Top"=w676) -> ()  [unwired: 1 in, 2 out]
                    }
                  }
                }
              }
            }
          }
        }
      }
    }
  }
  n328 = global write "GVSNew View Global.vi" "DataView_Global"(w6) -> ()
